vi "Get Channels from Line.vi"(11 "Line":T1) -> (3 "Channels":refnum<class "TBM channel.lvclass">[](array[class]))   [LabVIEW 2015, in "Increment configuration.lvclass"]
doc: "Returns an array of channels for a single line."
uses:
  Increment configuration.lvclass
  <vilib>/NI/Tag Bus Module Framework/channel/TBM channel.lvclass
  Line.ctl
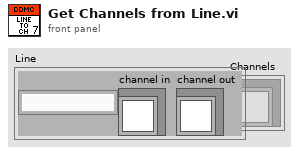
[diagram p1: front panel]
types:
  T1 = typedef "Increment configuration.lvclass/Line.ctl" = cluster{"Name":string, "channel in":refnum<class "TBM channel.lvclass">, "channel out":refnum<class "TBM channel.lvclass">}
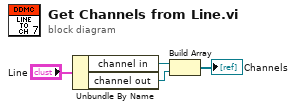
[diagram p0: block diagram]
diagram:
  n1 = Unbundle By Name("Line") -> ("channel in"=w2:refnum<class "TBM channel.lvclass">, "channel out"=w1:refnum<class "TBM channel.lvclass">)
  n2 = Build Array(w2, w1) -> (→"Channels":refnum<class "TBM channel.lvclass">[])
